vi "Get System Definition Ref.vi"(8 "error in (no error)":errorcluster, 11 "System Definition Path":path) -> (0 "error out":errorcluster, 2 "System Definition Root Ref":refnum<k24>, 3 "System Definition Ref":refnum<k24>)   [LabVIEW 2019, in "TLCD Test.lvclass"]
uses:
  TLCD Test.lvclass
  NationalInstruments.VeriStand.SystemDefinitionAPI
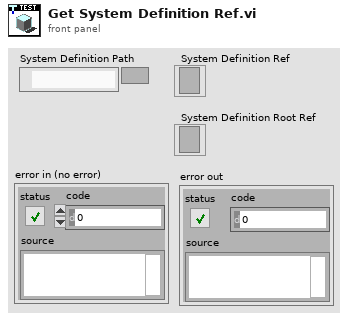
[diagram p1: front panel]
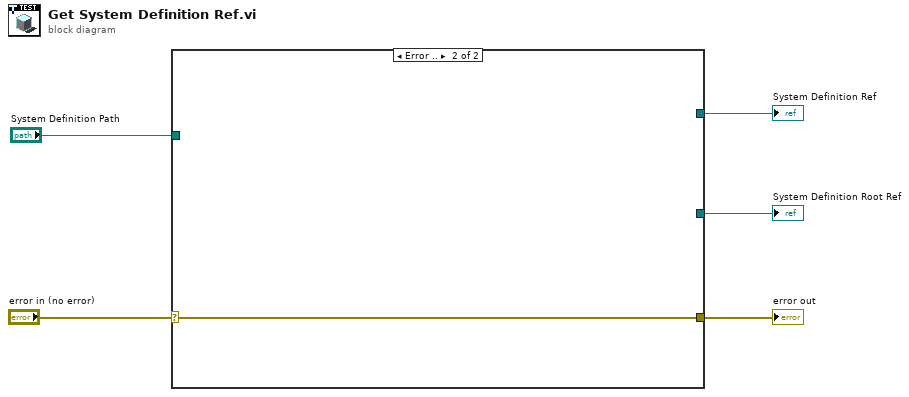
[diagram p0: block diagram]
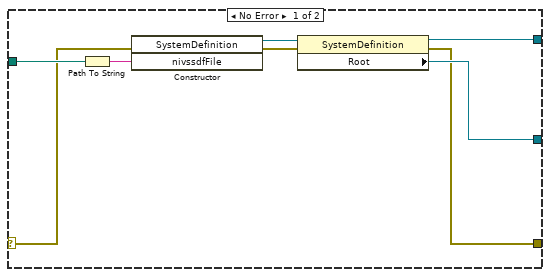
[diagram p2: hidden frame]
diagram:
  n1 = case shown="Error .." "error in (no error)" {
    selector: "error in (no error)" -> [w6 w14]
    tunnel: [w13 _] -> w5
    tunnel: "System Definition Path" -> [w12 _]
    tunnel: [w8 _] -> w3
    tunnel: [w7 w14] -> w2
    frame No Error {
      n2 = Path To String(path=w12) -> (string=w11:string)
      n3 = constructor class="SystemDefinition"(error in=w6, "nivssdfFile"=w11) -> (reference out=w9:refnum<k24>, error out=w10:errorcluster)  [unwired: 2 in, 2 out]
      n4 = property class="SystemDefinition"(reference=w9, error in=w10) -> (reference out=w13:refnum<k24>, error out=w7:errorcluster, "Root"=w8:refnum<k24>)
    }
    frame Error {
    }
  }
  "System Definition Ref" <- w5
  "System Definition Root Ref" <- w3
  "error out" <- w2
